vi "Write Component Root path.vi"(8 "error in (no error)":errorcluster, 10 "Component Definition ini path":path, 11 "Export in":refnum<class "Export.lvclass">) -> (0 "error out":errorcluster, 3 "Export out":refnum<class "Export.lvclass">)   [LabVIEW 2017, in "CL_G3_VIComponentBuilder.lvlib" / "Export.lvclass"]
uses:
  Export.lvclass
  Export.lvclass/Export.ctl
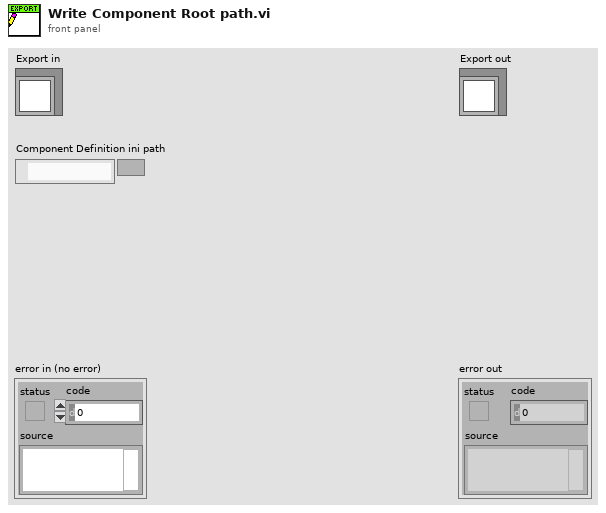
[diagram p1: front panel]
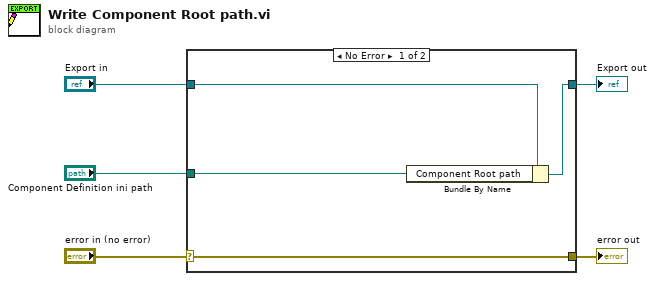
[diagram p0: block diagram]
diagram:
  n1 = case shown="No Error" "error in (no error)" {
    selector: "error in (no error)" -> [w9 w10]
    tunnel: [w9 w10] -> w4
    tunnel: [w7 w11] -> w2
    tunnel: "Export in" -> [w8 w11]
    tunnel: "Component Definition ini path" -> [w6 _]
    frame No Error {
      n2 = Bundle By Name(cluster=w8, "Component Root path"=w6) -> (w7:refnum<class "Export.lvclass">)
    }
    frame Error {
    }
  }
  "error out" <- w4
  "Export out" <- w2
